vi "Init.vi"(10 "String":string) -> (3 "xxxxx Msg Strategy out":refnum<class "xxxxx Msg Strategy.lvclass">)   [LabVIEW 2021, in "jettl Tools.lvlib" / "jettl Msg xxxxx.lvlib" / "xxxxx Msg Strategy.lvclass"]
uses:
  xxxxx Msg Strategy.lvclass
  xxxxx Msg Strategy.lvclass/xxxxx Msg Strategy.ctl
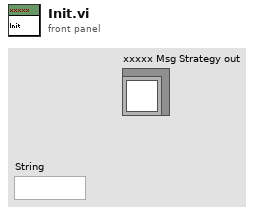
[diagram p1: front panel]
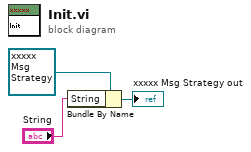
[diagram p0: block diagram]
diagram:
  n1 = Bundle By Name(cluster=refnum<class "xxxxx Msg Strategy.lvclass"> refnum ("xxxxx Msg Strategy out"), "String"="String") -> (→"xxxxx Msg Strategy out":refnum<class "xxxxx Msg Strategy.lvclass">)
